vi "Send Autosampler Status Update.vi"(7 "Message Priority (Normal)":T3=enum."Normal", 8 "error in (no error)":errorcluster, 10 "Autosampler Status":T1, 11 "Message Enqueuer":refnum<class "Message Enqueuer.lvclass">) -> (0 "error out":errorcluster, 3 "Message Enqueuer out":refnum<class "Message Enqueuer.lvclass">)   [LabVIEW 2023, in "Main Window.lvlib" / "Autosampler Status Update Msg.lvclass"]
doc: "This VI sends the message to an actor."
uses:
  Autosampler Status Update Msg.lvclass
  Autosampler Status Update Msg.lvclass/Autosampler Status Update Msg.ctl
  <vilib>/ActorFramework/Message Enqueuer/Message Enqueuer.lvclass
  <vilib>/ActorFramework/Message Enqueuer/Message Priority.ctl
  Hardware/Autosampler/Autosampler Status.ctl
  Hardware/Autosampler/Autosampler.lvlib
  Hardware/Autosampler/Autosampler State.ctl
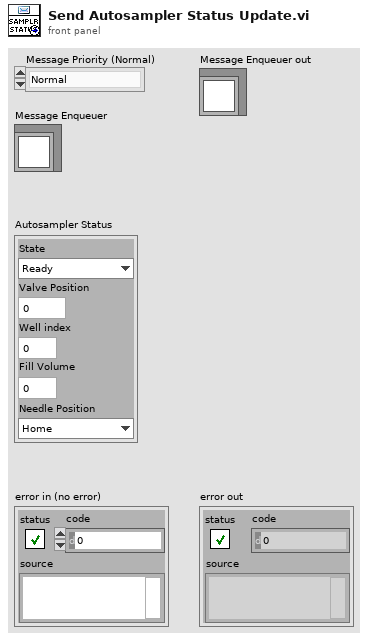
[diagram p1: front panel]
types:
  T1 = typedef "Autosampler.lvlib/Autosampler Status.ctl" = cluster{"State":T2, "Valve Position":u16, "Well index":u16, "Fill Volume":u16, "Needle Position":enum16{"Home", "Well", "Wash Port"}}
  T2 = typedef "Autosampler.lvlib/Autosampler State.ctl" = enum16{"Ready", "Injection", "Washing", "Shaking", "Getting Ready", "Error"}
  T3 = typedef "Actor Framework.lvlib/Message Enqueuer.lvclass/Message Priority.ctl" = enum16{"Low", "Normal", "High"}
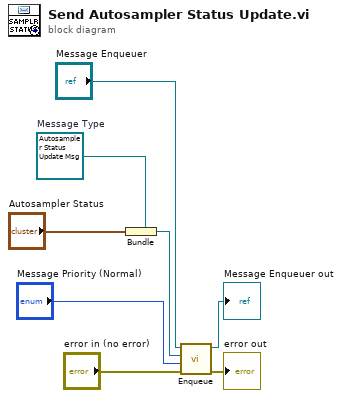
[diagram p0: block diagram]
diagram:
  w2 = refnum<class "Autosampler Status Update Msg.lvclass"> refnum  # Message Type
  n1 = Bundle(cluster=w2, "Autosampler Status") -> (w3:refnum<class "Autosampler Status Update Msg.lvclass">)
  n2 = call <vilib>:"Enqueue.vi"("error in (no error)"="error in (no error)", "Message Priority (Normal)"="Message Priority (Normal)", "Message"=w3, "Message Enqueuer in"="Message Enqueuer") -> ("error out"=→"error out":errorcluster, "Message Enqueuer out"=→"Message Enqueuer out":refnum<class "Message Enqueuer.lvclass">)  [unwired: 6 in]
